vi "Condition.vi"(8 "error in (no error)":errorcluster, 11 "Measurement2D in":refnum<class "Measurement2D.lvclass">) -> (0 "error out":errorcluster, 2 "Finish?":bool, 3 "Measurement2D out":refnum<class "Measurement2D.lvclass">)   [LabVIEW 2014, in "Measurement2D.lvclass"]
uses:
  Measurement2D.lvclass
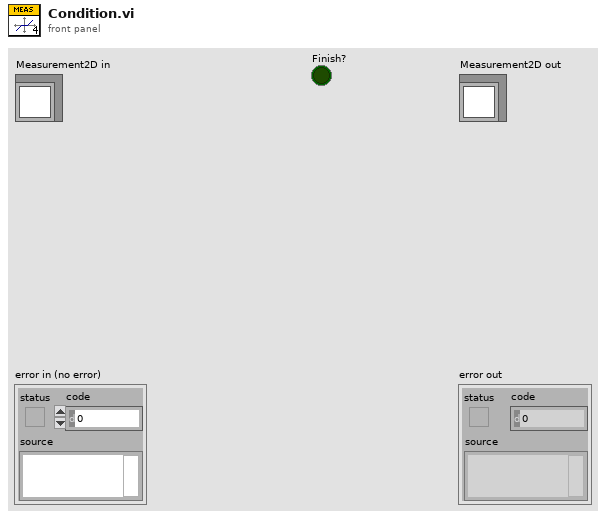
[diagram p1: front panel]
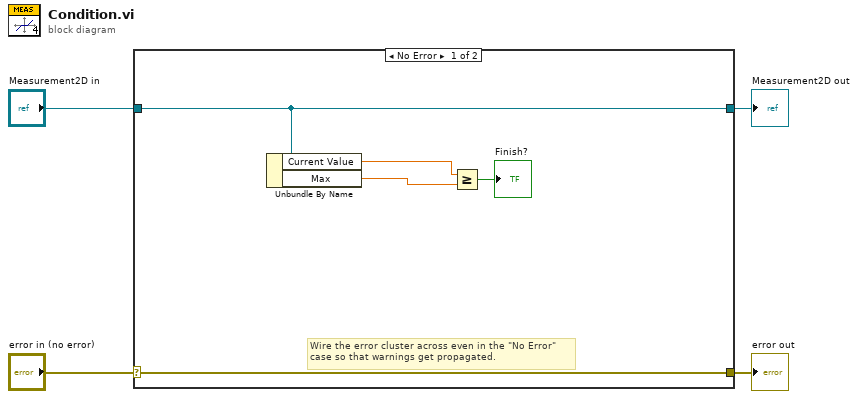
[diagram p0: block diagram]
diagram:
  n1 = case shown="No Error" "error in (no error)" {
    selector: "error in (no error)" -> [w9 w11]
    tunnel: [w9 w11] -> w3
    tunnel: [w8 w10] -> w1
    tunnel: "Measurement2D in" -> [w8 w10]
    frame No Error {
      # "Wire the error cluster across even in the \"No Error\"\ncase so that warnings get propagated."
      n2 = Unbundle By Name(w8) -> ("Current Value"=w7:dbl, "Max"=w6:dbl)
      n3 = Greater Or Equal?(x=w7, y=w6) -> (x >= y?=→"Finish?":bool)
    }
    frame Error {
    }
  }
  "error out" <- w3
  "Measurement2D out" <- w1
